vi "SLMServer.vi"() -> ()   [LabVIEW 2013, in "SLMServer.lvlib"]
uses:
  SLMServer.lvlib
  Sources/Supported-module-types.ctl
  Sources/Settings.ctl
  Sources/SLMServer.lvclass
panel:
  in  "Exit all clients":bool
  out "Activity log":string[](array[string])
  out "Active clients":T1(array[cluster]) {"ID" format="%010d"}
  in  "Start new client":bool
  in  "Select module":T2
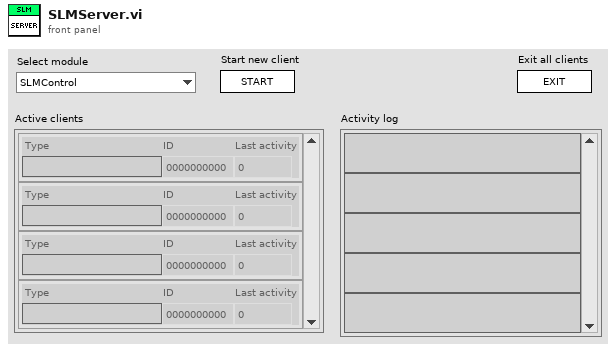
[diagram p1: front panel]
types:
  T1 = cluster{"Type":string, "ID":i32, "Last activity":i32}[]
  T2 = typedef "SLMServer.lvlib/SLMServer.lvclass/Supported-module-types.ctl" = enum16{"SLMControl", "PowderDeposition", "CameraVision", "Server", "All", "StrategyParser", "MaterialCharacterization", "StatusMonitor", "SLMSimulation", "LaserCharacterization"}
  T3 = typedef "SLMServer.lvlib/SLMServer.lvclass/Settings.ctl" = cluster{"Client settings":cluster{"Module type":T2, "MaxClients":i32, "Path":path, "Relative path?":bool}[], "Max backlog entries":i32, "Heartbeat timeout":dbl}
  T4 = typedef "SLMServer.lvlib/SLMServer.lvclass/Object-reference.ctl" = refnum<data-value>
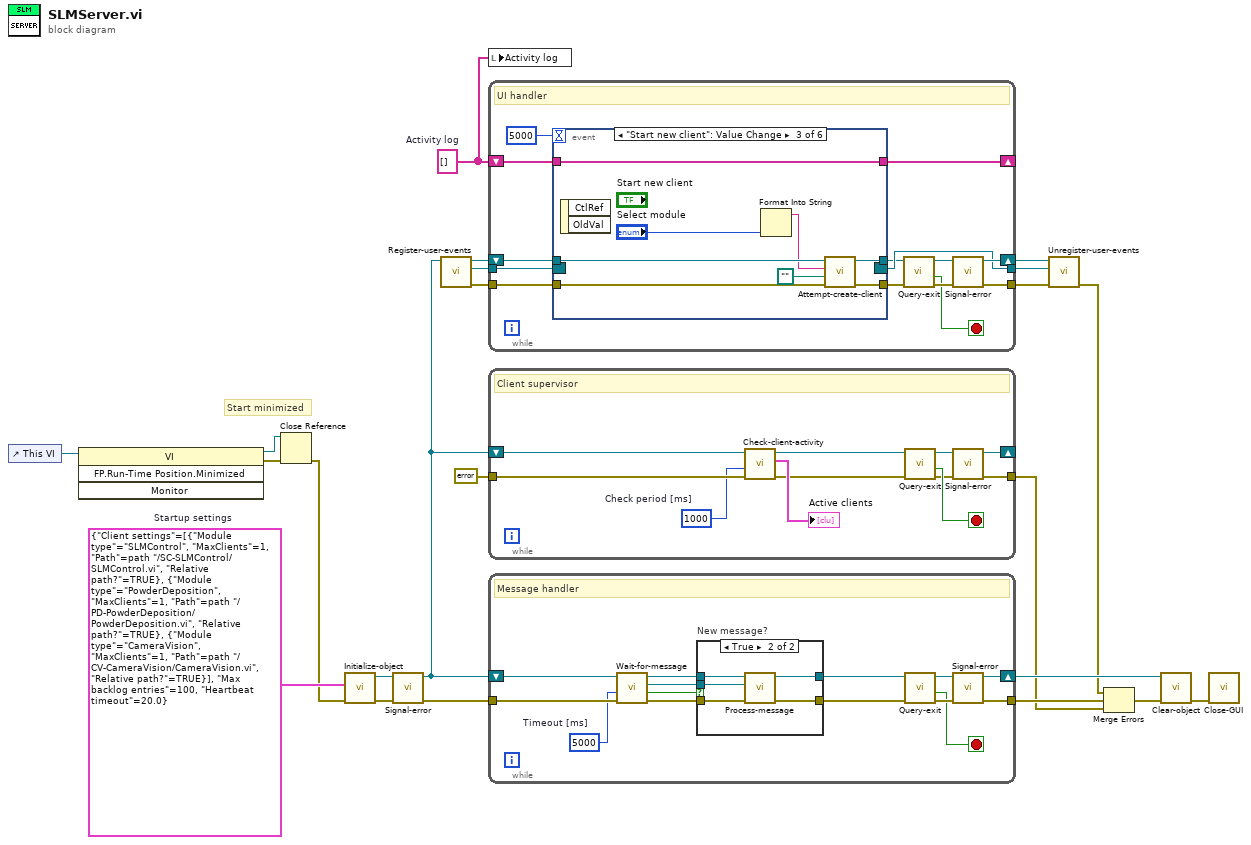
[diagram p0: block diagram]
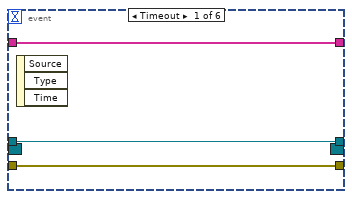
[diagram p2: hidden frame]
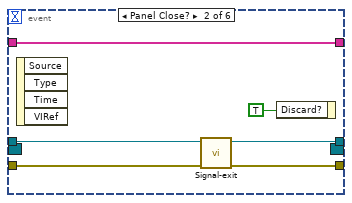
[diagram p3: hidden frame]
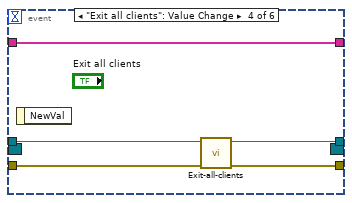
[diagram p4: hidden frame]
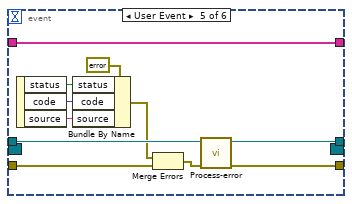
[diagram p5: hidden frame]
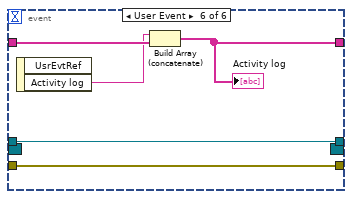
[diagram p6: hidden frame]
diagram:
  w11 = string[] []  # Activity log
  w23 = T3 {"Client settings"=[{"Module type"=enum."SLMControl", "MaxClients"=1, "Path"=path "../SC-SLMControl/SLMControl.vi", "Relative path?"=TRUE}, {"Module type"=enum."PowderDeposition", "MaxClients"=1, "Path"=path "../PD-PowderDeposition/PowderDeposition.vi", "Relative path?"=TRUE}, {"Module type"=enum."CameraVision", "MaxClients"=1, "Path"=path "../CV-CameraVision/CameraVision.vi", "Relative path?"=TRUE}], "Max backlog entries"=100, "Heartbeat timeout"=20.0}  # Startup settings
  # "Start minimized"
  n1 = control-ref of="This VI"() -> (w10:refnum<vi>)
  n2 = invoke class="VI" method="FP.Run-Time Position.Minimized"(reference=w10) -> (reference out=w8:refnum<vi>, error out=w9:errorcluster)  [unwired: 3 in, 2 out]
  n3 = Close Reference(reference=w8, error in (no error)=w9) -> (error out=w7:errorcluster)
  n4 = call "Initialize-object.vi"("error in (no error)"=w7, "Settings"=w23) -> ("error out"=w2:errorcluster, "Reference out"=w4:T4)  [unwired: 8 in]
  n5 = call "Signal-error.vi"("error in (no error)"=w2, "ModComm in"=w4) -> ("error out"=w1:errorcluster, "ModComm out"=w3:T4)  [unwired: 8 in]
  n6 = call "Register-user-events.vi"("ModComm in"=w3) -> ("error out"=w17:errorcluster, "Event Registration"=w16:refnum<event-registration>, "ModComm out"=w18:T4)  [unwired: 8 in]
  n7 = local write "Activity log"(w11) -> ()
  n8 = while {
    shift-right: [w33] -> w15
    shift-left: w18 -> [w24]
    tunnel: w16 -> [w36]
    shift-right: [w34] -> _
    shift-left: w11 -> [w35]
    tunnel: [w32] -> w12
    tunnel: w17 -> [w37]
    tunnel: [w31] -> w14
    stop <- w27 stop-if-true
    # "UI handler"
    n9 = event shown="[2] \"Start new client\": Value Change" {
      selector: w36 -> [_ _ _ _ _ _]
      dyn-events: [_ _ _ _ _ _] -> w32
      timeout: 5000 -> [_ _ _ _ _ _]
      tunnel: w24 -> [w40 w45 w53 w59 w66 w75]
      tunnel: [w40 w44 w52 w57 w65 w75] -> w25
      tunnel: w37 -> [w39 w43 w50 w56 w62 w74]
      tunnel: [w39 w42 w51 w55 w61 w74] -> w29
      tunnel: w35 -> [w38 w41 w54 w58 w60 w73]
      tunnel: [w38 w41 w54 w58 w60 w71] -> w34
      event Timeout {
        n10 = event-data() -> ()  [unwired: 1 in, 3 out]
      }
      event Panel Close? {
        n11 = event-data() -> ()  [unwired: 1 in, 4 out]
        n12 = call "Signal-exit.vi"("error in (no error)"=w43, "ModComm in"=w45) -> ("error out"=w42:errorcluster, "ModComm out"=w44:T4)  [unwired: 8 in]
        n13 = event-data("Discard?"=TRUE) -> ()  [unwired: 1 in, 1 out]
      }
      event "Start new client": Value Change {
        n14 = event-data() -> ()  [unwired: 1 in, 2 out]
        n15 = Format Into String("Select module") -> (resulting string=w48:string)  [unwired: 3 in, 1 out]
        n16 = call "Attempt-create-client.vi"("error in (no error)"=w50, "Module path"=path "", "Module type"=w48, "ModComm in"=w53) -> ("error out"=w51:errorcluster, "ModComm out"=w52:T4)  [unwired: 6 in]
      }
      event "Exit all clients": Value Change {
        n17 = event-data() -> ()  [unwired: 1 in, 1 out]
        n18 = call "Exit-all-clients.vi"("error in (no error)"=w56, "ModComm in"=w59) -> ("error out"=w55:errorcluster, "ModComm out"=w57:T4)  [unwired: 8 in]
      }
      event User Event {
        n19 = event-data() -> ("status"=w69:bool, "code"=w68:i32, "source"=w67:string)  [unwired: 1 in]
        n20 = Bundle By Name(cluster=errorcluster {"status"=FALSE, "code"=0, "source"=""} ("error constant"), "status"=w69, "code"=w68, "source"=w67) -> (w63:errorcluster)
        n21 = Merge Errors(w63, w62) -> (w64:errorcluster)
        n22 = call "Process-error.vi"("error in (no error)"=w64, "ModComm in"=w66) -> ("error out"=w61:errorcluster, "ModComm out"=w65:T4)  [unwired: 8 in]
      }
      event User Event {
        n23 = event-data() -> ("Activity log"=w72:string)  [unwired: 1 in, 1 out]
        n24 = Build Array (concatenate)(w72, w73) -> (w71:string[])
        "Activity log" <- w71
      }
    }
    n25 = call "Query-exit.vi"("error in (no error)"=w29, "ModComm in"=w25) -> ("error out"=w28:errorcluster, "Exit?"=w27:bool, "ModComm out"=w30:T4)  [unwired: 7 in]
    n26 = call "Signal-error.vi"("error in (no error)"=w28, "ModComm in"=w30) -> ("error out"=w31:errorcluster, "ModComm out"=w33:T4)  [unwired: 8 in]
  }
  n27 = while {
    shift-right: [w80] -> _
    shift-left: w3 -> [w85]
    tunnel: errorcluster {"status"=FALSE, "code"=0, "source"=""} ("error constant") -> [w84]
    tunnel: [w81] -> w19
    stop <- w86 stop-if-true
    w79 = u32 1000  # Check period [ms]
    # "Client supervisor"
    n28 = call "Check-client-activity.vi"("error in (no error)"=w84, "Check period"=w79, "ModComm in"=w85) -> ("error out"=w76:errorcluster, "Active clients"=→"Active clients":T1, "ModComm out"=w77:T4)  [unwired: 6 in]
    n29 = call "Query-exit.vi"("error in (no error)"=w76, "ModComm in"=w77) -> ("error out"=w82:errorcluster, "Exit?"=w86:bool, "ModComm out"=w83:T4)  [unwired: 7 in]
    n30 = call "Signal-error.vi"("error in (no error)"=w82, "ModComm in"=w83) -> ("error out"=w81:errorcluster, "ModComm out"=w80:T4)  [unwired: 8 in]
  }
  n31 = while {
    shift-right: [w90] -> w22
    shift-left: w3 -> [w100]
    tunnel: w1 -> [w99]
    tunnel: [w89] -> w21
    stop <- w87 stop-if-true
    w98 = 5000  # Timeout [ms]
    # "Message handler"
    n32 = call "Wait-for-message.vi"("error in (no error)"=w99, "Timeout"=w98, "ModComm in"=w100) -> ("error out"=w95:errorcluster, "New message?"=w97:bool, "Message"=w88:refnum<class "Message.lvclass">, "ModComm out"=w96:T4)  [unwired: 5 in]
    n33 = case "New message?" shown="True" w97 {
      tunnel: w96 -> [w102 w107]
      tunnel: w95 -> [w101 w106]
      tunnel: w88 -> [_ w105]
      tunnel: [w101 w104] -> w93
      tunnel: [w102 w103] -> w94
      frame False {
      }
      frame True {
        n34 = call "Process-message.vi"("error in (no error)"=w106, "Message"=w105, "ModComm in"=w107) -> ("error out"=w104:errorcluster, "ModComm out"=w103:T4)  [unwired: 7 in]
      }
    }
    n35 = call "Query-exit.vi"("error in (no error)"=w93, "ModComm in"=w94) -> ("error out"=w92:errorcluster, "Exit?"=w87:bool, "ModComm out"=w91:T4)  [unwired: 7 in]
    n36 = call "Signal-error.vi"("error in (no error)"=w92, "ModComm in"=w91) -> ("error out"=w89:errorcluster, "ModComm out"=w90:T4)  [unwired: 8 in]
  }
  n37 = call "Unregister-user-events.vi"("error in (no error)"=w14, "Event Registration"=w12, "ModComm in"=w15) -> ("error out"=w13:errorcluster)  [unwired: 7 in, 1 out]
  n38 = Merge Errors(w13, w21, w19) -> (w20:errorcluster)
  n39 = call "Clear-object.vi"("error in (no error)"=w20, "Reference in"=w22) -> ("error out"=w5:errorcluster)  [unwired: 9 in]
  n40 = call "Close-GUI.vi"("error in (no error)"=w5) -> ()  [unwired: 10 in, 1 out]
